vi "Check Target LV Package Version.vi"(8 "Error In":errorcluster, 11 "Install LV Data":T1={"SSH Session"=refnum, "Status Log"="", "Detailed Log"="", "Credentials"={"Hostname or IP"="192.168.7.2", "Username"="root", "Password"=""}, "Target Info"={"OS Version"="", "CPU"="", "Systemd Version"="", "Internet Access"=FALSE, "Device Type"="", "LV Installed Ver"="", "LV Available Ver"="", "LV Upgrade Available"=FALSE, "Hostname"="", "NIC Info"=[]}, "Reboot Required?"=FALSE}) -> (0 "Error Out":errorcluster, 1 "Available Version":string, 2 "Installed Version":string, 3 "Install LV Data":T1={"SSH Session"=refnum, "Status Log"="", "Detailed Log"="", "Credentials"={"Hostname or IP"="192.168.7.2", "Username"="root", "Password"=""}, "Target Info"={"OS Version"="", "CPU"="", "Systemd Version"="", "Internet Access"=FALSE, "Device Type"="", "LV Installed Ver"="", "LV Available Ver"="", "LV Upgrade Available"=FALSE, "Hostname"="", "NIC Info"=[]}, "Reboot Required?"=FALSE}, 4 "Upgrade Available?":bool)   [LabVIEW 2014, in "LMH-LINX.lvlib"]
uses:
  <vilib>/MakerHub/LINX/LMH-LINX.lvlib
  <vilib>/MakerHub/LINX/Private/Utilties/Target Management/Install LV Data.ctl
  C:/Program Files (x86)/National Instruments/LabVIEW 2014/vi.lib/MakerHub/LINX/Resources/Renci.SshNet.dll
  Resources/Renci.SshNet.dll
  <vilib>/MakerHub/LINX/Private/Utilties/Target Management/Target Info.ctl
  <vilib>/MakerHub/LINX/Private/Utilties/Target Management/NIC Info.ctl
  <vilib>/MakerHub/LINX/Private/Utilties/Target Management/NIC Mode.ctl
  <vilib>/regexp/Match Regular Expression.xnode
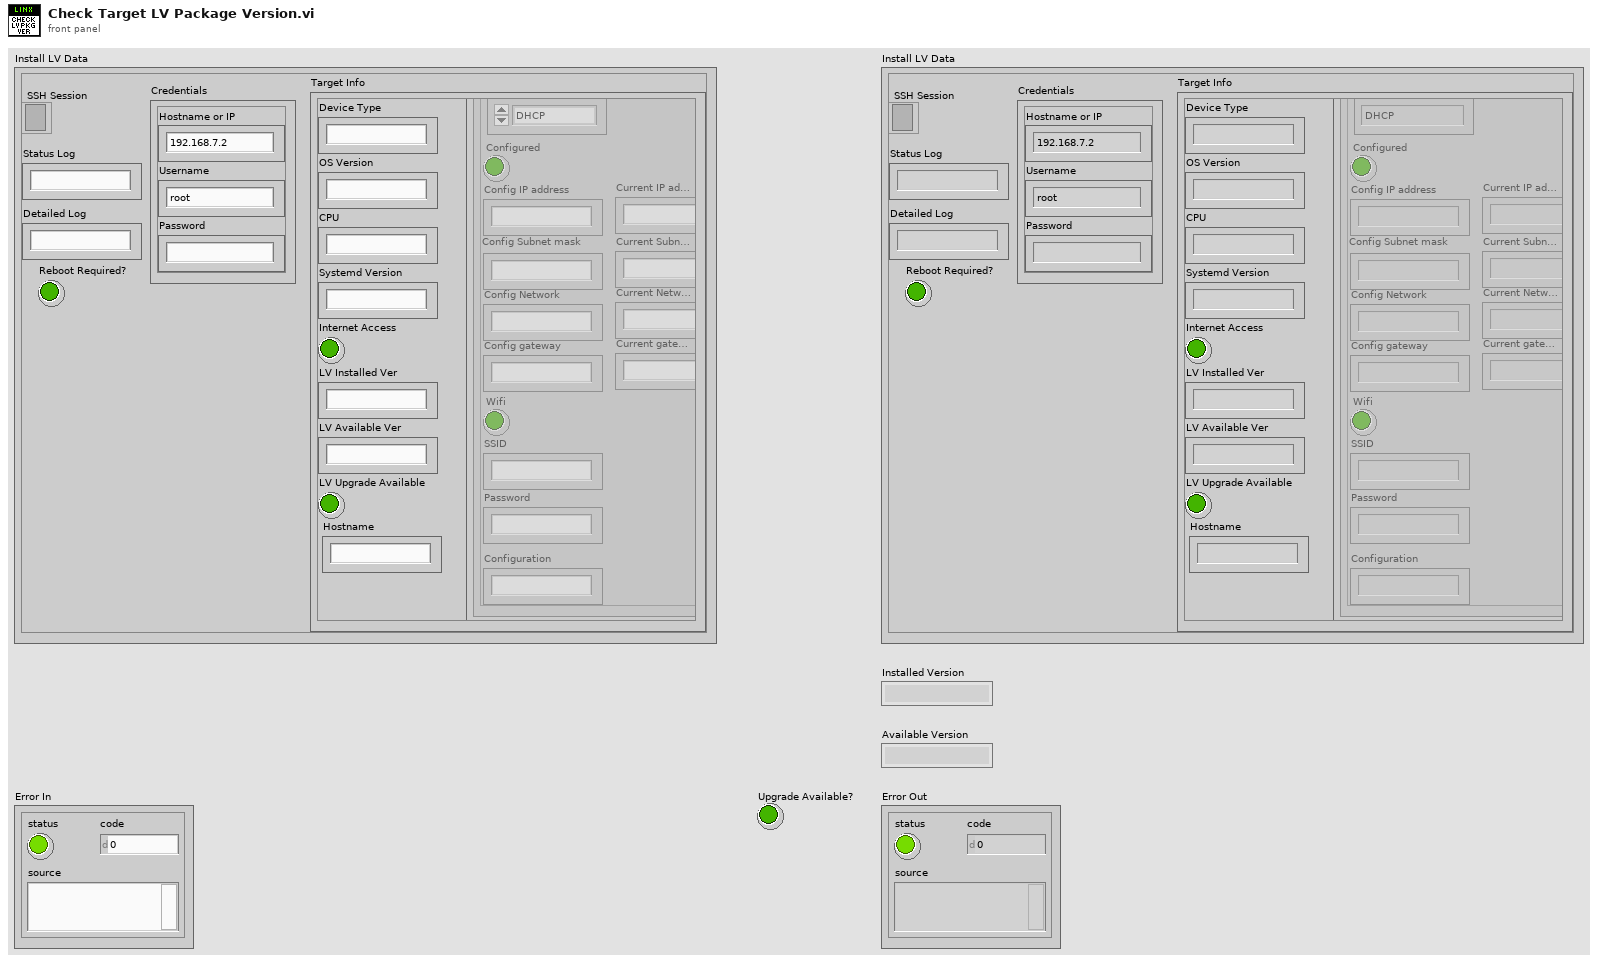
[diagram p1: front panel]
types:
  T1 = typedef "LMH-LINX.lvlib/Install LV Data.ctl" = cluster{"SSH Session":refnum<k24>, "Status Log":string, "Detailed Log":string, "Credentials":cluster{"Hostname or IP":string, "Username":string, "Password":string}, "Target Info":T2, "Reboot Required?":bool}
  T2 = typedef "LMH-LINX.lvlib/Target Info.ctl" = cluster{"OS Version":string, "CPU":string, "Systemd Version":string, "Internet Access":bool, "Device Type":string, "LV Installed Ver":string, "LV Available Ver":string, "LV Upgrade Available":bool, "Hostname":string, "NIC Info":T3[]}
  T3 = typedef "LMH-LINX.lvlib/NIC Info.ctl" = cluster{"Name":string, "NIC Mode":T4, "Configured":bool, "Config IP address":string, "Config Subnet mask":string, "Config Network":string, "Config gateway":string, "Wifi":bool, "SSID":string, "Password":string, "Configuration":string, "Current IP address":string, "Current Subnet mask":string, "Current gateway":string, "Current Network":string}
  T4 = typedef "LMH-LINX.lvlib/NIC Mode.ctl" = enum16{"DHCP", "Static", "Loopback"}
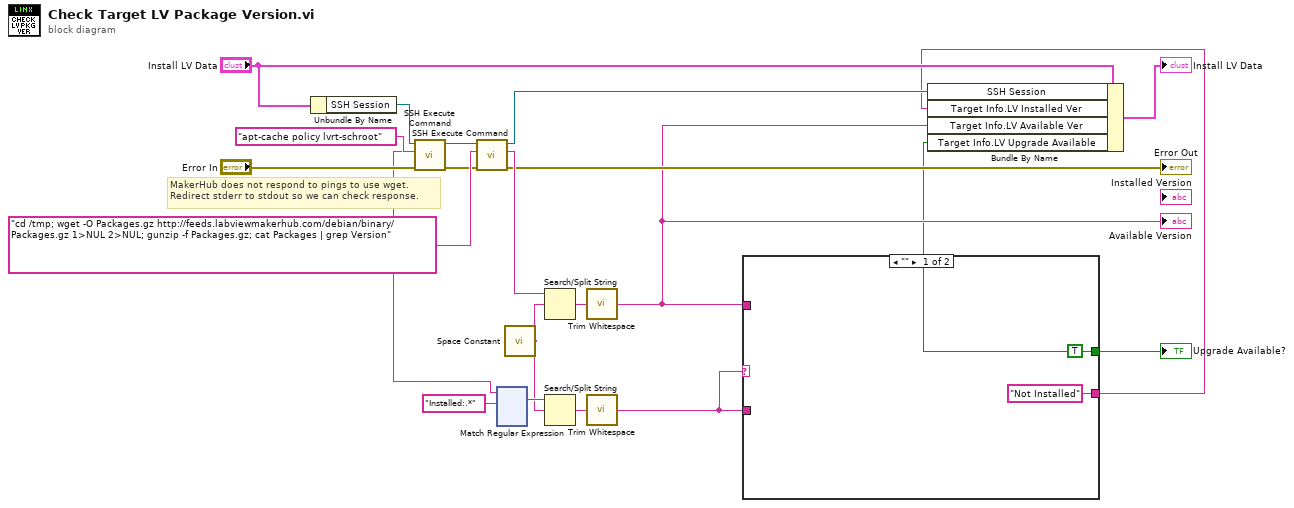
[diagram p0: block diagram]
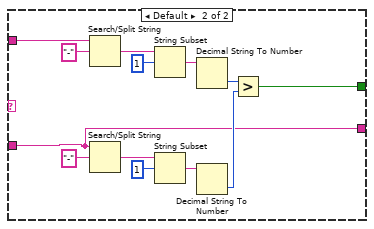
[diagram p2: hidden frame]
diagram:
  # "MakerHub does not respond to pings to use wget.\nRedirect stderr to stdout so we can check response."
  n1 = Unbundle By Name("Install LV Data") -> ("SSH Session"=w20:refnum<k24>)
  n2 = call <vilib>:"SSH Execute Command.vi"("Error In"="Error In", "Command"="apt-cache policy lvrt-schroot", "SSH Session"=w20) -> ("Error Out"=w9:errorcluster, "Std Out"=w11:string, "SSH Session"=w8:refnum<k24>)  [unwired: 6 in]
  n3 = call <vilib>:"SSH Execute Command.vi"("Error In"=w9, "Command"="cd /tmp; wget -O Packages.gz http://feeds.labviewmakerhub.com/debian/binary/Packages.gz 1>NUL 2>NUL; gunzip -f Packages.gz; cat Packages | grep Version", "SSH Session"=w8) -> ("Error Out"=→"Error Out":errorcluster, "Std Out"=w6:string, "SSH Session"=w7:refnum<k24>)  [unwired: 6 in]
  n4 = xnode "Match Regular Expression"("input string"=w11, "regular expression"="Installed:.*") -> ("whole match"=w15:string)  [unwired: 4 in, 4 out]
  n5 = call <vilib>:"Space Constant.vi"() -> ("String"=w12:string)
  n6 = Search/Split String(string=w6, search string/char (-)=w12) -> (match + rest of string=w13:string)  [unwired: 1 in, 2 out]
  n7 = Search/Split String(string=w15, search string/char (-)=w12) -> (match + rest of string=w14:string)  [unwired: 1 in, 2 out]
  n8 = call <vilib>:"Trim Whitespace.vi"("string"=w13) -> ("trimmed string"=w4:string)  [unwired: 1 in]
  "Available Version" <- w4
  n9 = call <vilib>:"Trim Whitespace.vi"("string"=w14) -> ("trimmed string"=w1:string)  [unwired: 1 in]
  n10 = case shown="\"\"" w1 {
    tunnel: w1 -> [_ w24]
    tunnel: w4 -> [_ w26]
    tunnel: [TRUE w25] -> w3
    tunnel: ["Not Installed" ("trimmed string") w24] -> w2
    frame "" {
    }
    frame Default {
      n11 = Search/Split String(string=w26, search string/char (-)="-") -> (match + rest of string=w28:string)  [unwired: 1 in, 2 out]
      n12 = Search/Split String(string=w24, search string/char (-)="-") -> (match + rest of string=w27:string)  [unwired: 1 in, 2 out]
      n13 = String Subset(string=w28, offset (0)=1) -> (substring=w31:string)  [unwired: 1 in]
      n14 = String Subset(string=w27, offset (0)=1) -> (substring=w29:string)  [unwired: 1 in]
      n15 = Decimal String To Number(string=w31) -> (number=w34:i32)  [unwired: 2 in, 1 out]
      n16 = Decimal String To Number(string=w29) -> (number=w33:i32)  [unwired: 2 in, 1 out]
      n17 = Greater?(x=w34, y=w33) -> (0:w25:bool)
    }
  }
  "Upgrade Available?" <- w3
  n18 = Bundle By Name(cluster="Install LV Data", "SSH Session"=w7, "Target Info.LV Installed Ver"=w2, "Target Info.LV Available Ver"=w4, "Target Info.LV Upgrade Available"=w3) -> (→"Install LV Data":T1)
